vi "Keithley2200series_2_dose.vi"() -> ()   [LabVIEW 2010]
uses:
  <vilib>/Utility/file.llb/Write To Spreadsheet File (string).vi
  C:/Users/rad/Desktop/Keithley 2200 Series Power Supplies Ver 1.2 (LV2009)/Keithley 2200 Series/Keithley 2200 Series.lvlib
panel:
  in  "millisecond multiple":u32
  out "Время,с":dbl
  in  "SEE th 2":dbl
  in  "SEE th 1":dbl
  in  "+ИП2":bool
  out "MEAS 2":string
  in  "Cml set 2":dbl
  in  "Function(0:Voltage) 3":u16(ring) items=["Voltage", "Current"]
  in  "Out set 2":dbl
  in  "VISA resource name 2":refnum<visa-resource-name>
  in  "Cml set":dbl
  in  "Function(0:Voltage) 2":u16(ring) items=["Voltage", "Current"]
  in  "Out set":dbl
  in  "Файл записи замеров":path
  out "MEAS":string
  in  "VISA resource name":refnum<visa-resource-name>
  in  "stop":bool
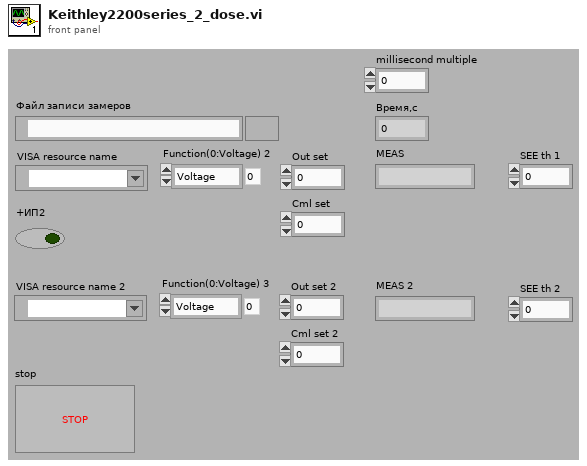
[diagram p1: front panel]
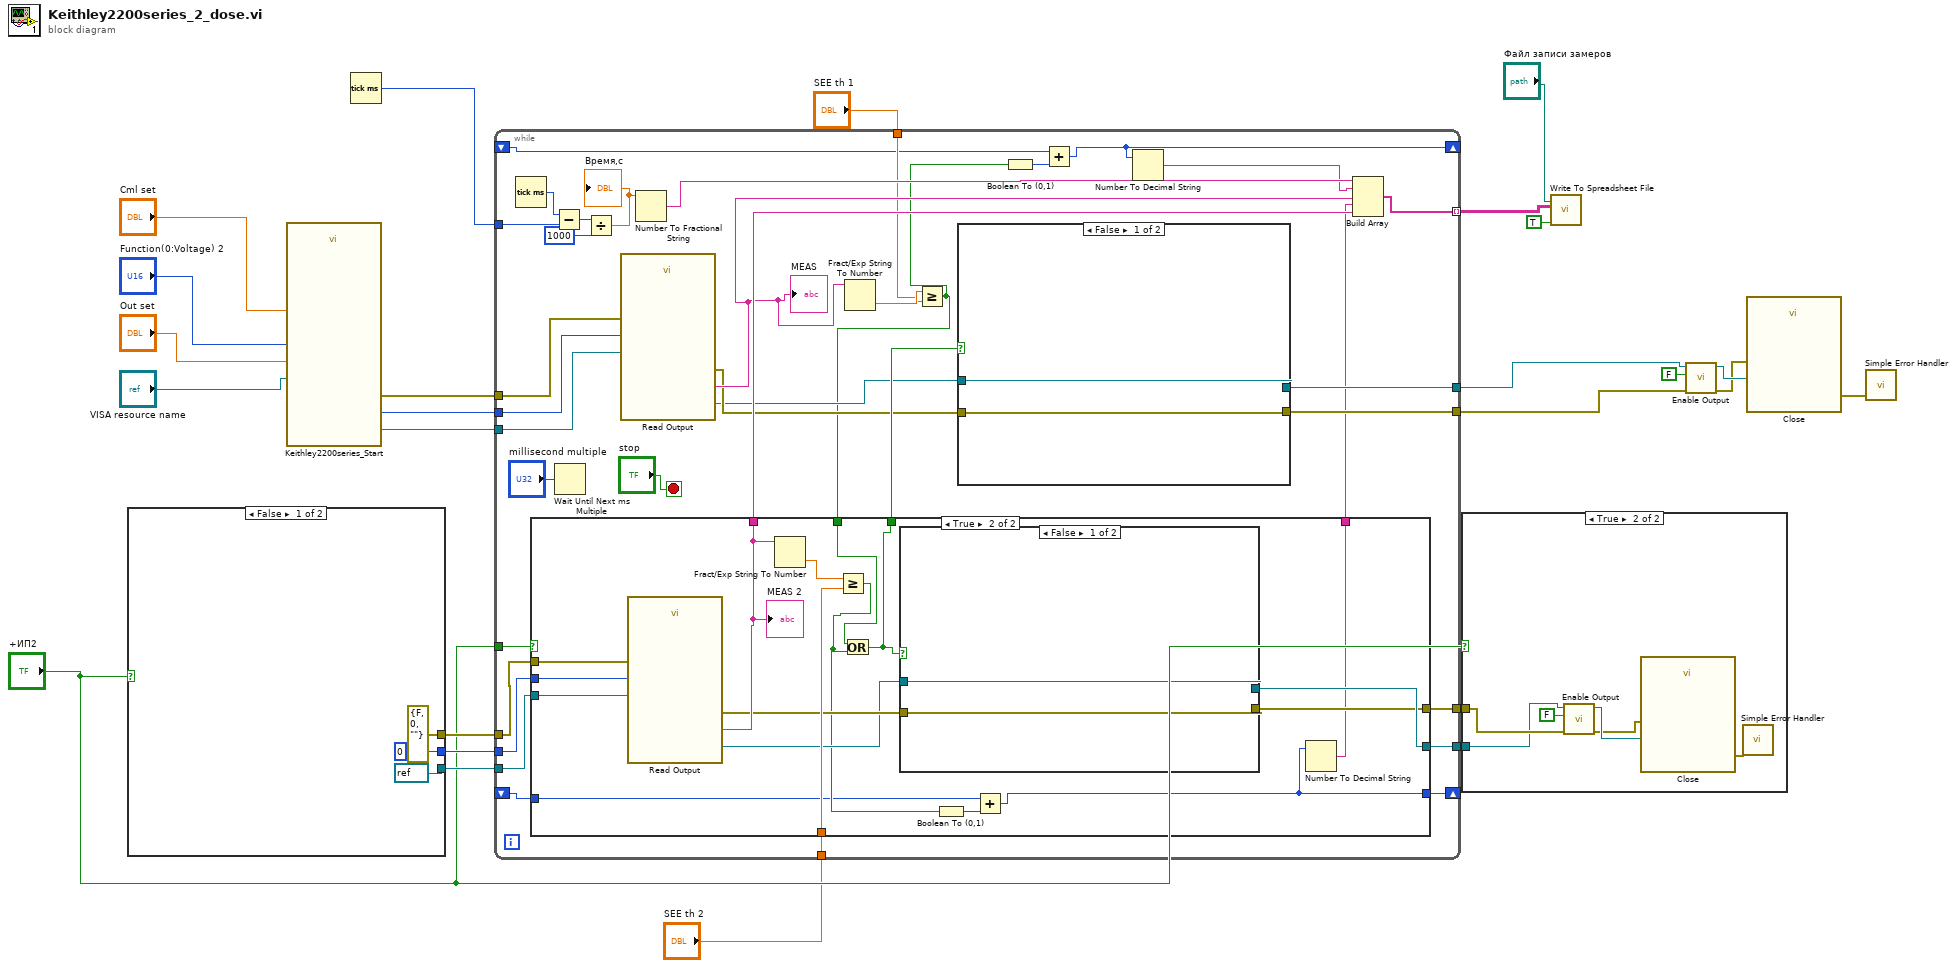
[diagram p0: block diagram]
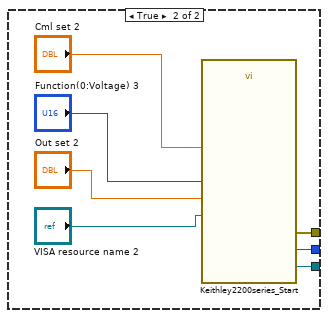
[diagram p3: hidden frame]
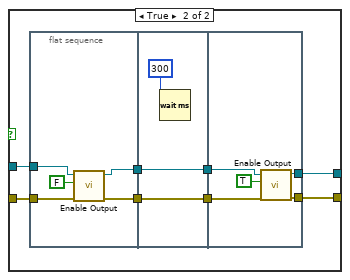
[diagram p4: hidden frame]
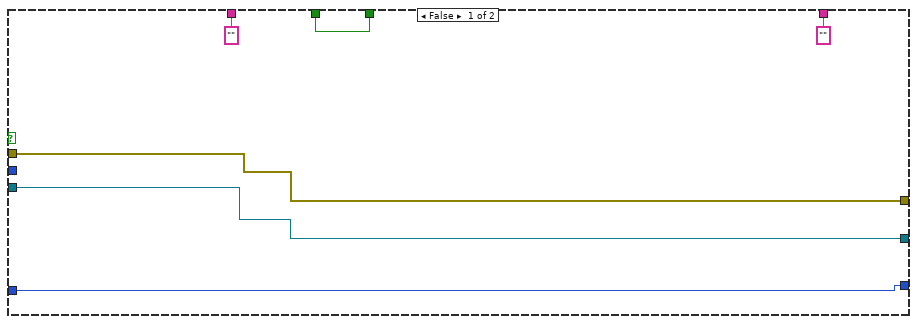
[diagram p5: hidden frame]
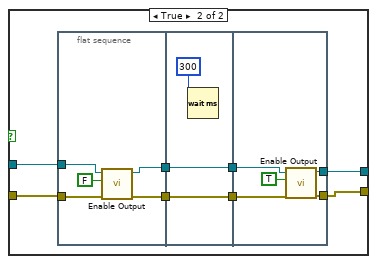
[diagram p6: hidden frame]
diagram:
  n1 = case shown="False" "+ИП2" {
    tunnel: [errorcluster {"status"=FALSE, "code"=0, "source"=""} ("error out 2") w31] -> w12
    tunnel: [0 ("Meas Func") w30] -> w11
    tunnel: [refnum<visa-resource-name> refnum ("VISA out") w29] -> w10
    frame False {
    }
    frame True {
      n2 = call "Keithley2200series_Start.vi"("VISA resource name 2"="VISA resource name 2", "Function(0:Voltage) 3"="Function(0:Voltage) 3", "Out set 2"="Out set 2", "Cml set 2"="Cml set 2") -> ("VISA out"=w29:refnum<visa-resource-name>, "Meas Func"=w30:i32, "error out 2"=w31:errorcluster)  [unwired: 1 in]
    }
  }
  n3 = call "Keithley2200series_Start.vi"("VISA resource name 2"="VISA resource name", "Function(0:Voltage) 3"="Function(0:Voltage) 2", "Out set 2"="Out set", "Cml set 2"="Cml set") -> ("VISA out"=w18:refnum<visa-resource-name>, "Meas Func"=w17:i32, "error out 2"=w16:errorcluster)  [unwired: 1 in]
  n4 = Tick Count (ms)() -> (millisecond timer value=w25:u32)
  n5 = while {
    tunnel: w25 -> [w70]
    tunnel: [w44] -> w24 mode=indexing
    tunnel: w18 -> [w65]
    tunnel: w17 -> [w64]
    tunnel: w16 -> [w63]
    tunnel: [w61] -> w14
    tunnel: [w60] -> w13
    tunnel: w12 -> [w59]
    tunnel: w11 -> [w58]
    tunnel: w10 -> [w57]
    tunnel: "+ИП2" -> [w56]
    tunnel: "SEE th 1" -> [w52]
    tunnel: "SEE th 2" -> [w51]
    tunnel: [w47] -> w3
    tunnel: [w46] -> w2
    shift-right: [w41] -> _
    shift-left: _ -> [w43]
    shift-right: [w38] -> _
    shift-left: _ -> [w39]
    stop <- "stop" stop-if-true
    n6 = Tick Count (ms)() -> (millisecond timer value=w71:u32)
    n7 = Subtract(x=w71, y=w70) -> (x-y=w68:u32)
    n8 = Wait Until Next ms Multiple(millisecond multiple="millisecond multiple") -> ()  [unwired: 1 out]
    n9 = Divide(x=w68, y=u32 1000) -> (x/y=w66:dbl)
    "Время,с" <- w66
    n10 = call "Read Output.vi"("VISA resource name"=w65, "Measurement Function (0:Voltage)"=w64, "error in (no error)"=w63) -> ("VISA resource name out"=w48:refnum<visa-resource-name>, "Measurement"=w54:string, "error out"=w49:errorcluster)  [unwired: 10 in]
    "MEAS" <- w54
    n11 = Number To Fractional String(number=w66) -> (F-format string=w69:string)  [unwired: 3 in]
    n12 = Fract/Exp String To Number(string=w54) -> (number=w53:dbl)  [unwired: 3 in, 1 out]
    n13 = Greater Or Equal?(x=w53, y=w52) -> (x >= y?=w42:bool)
    n14 = case shown="True" w56 {
      tunnel: [w100 w106] -> w61
      tunnel: [w99 w107] -> w60
      tunnel: ["" ("Measurement") w114] -> w55
      tunnel: w59 -> [w100 w117]
      tunnel: w58 -> [_ w116]
      tunnel: w57 -> [w99 w115]
      tunnel: w51 -> [_ w113]
      tunnel: w42 -> [w97 w111]
      tunnel: [w97 w110] -> w50
      tunnel: w39 -> [w96 w103]
      tunnel: [w96 w102] -> w38
      tunnel: ["" w101] -> w37
      frame False {
      }
      frame True {
        n15 = call "Read Output.vi"("VISA resource name"=w115, "Measurement Function (0:Voltage)"=w116, "error in (no error)"=w117) -> ("VISA resource name out"=w108:refnum<visa-resource-name>, "Measurement"=w114:string, "error out"=w109:errorcluster)  [unwired: 10 in]
        "MEAS 2" <- w114
        n16 = Fract/Exp String To Number(string=w114) -> (number=w112:dbl)  [unwired: 3 in, 1 out]
        n17 = Greater Or Equal?(x=w112, y=w113) -> (x >= y?=w104:bool)
        n18 = Or(x=w111, y=w104) -> (x .or. y?=w110:bool)
        n19 = case shown="False" w110 {
          tunnel: w109 -> [w118 w123]
          tunnel: w108 -> [w119 w122]
          tunnel: [w119 w121] -> w107
          tunnel: [w118 w120] -> w106
          frame False {
          }
          frame True {
            n20 = flat-sequence {
              tunnel: w123 -> [w131]
              tunnel: w122 -> [w130]
              tunnel: [w129] -> w127
              tunnel: [w128] -> w126
              tunnel: [w134] -> w125
              tunnel: w127 -> [w134]
              tunnel: [w133] -> w124
              tunnel: w126 -> [w133]
              tunnel: w125 -> [w139]
              tunnel: w124 -> [w138]
              tunnel: [w137] -> w121
              tunnel: [w136] -> w120
              frame #0 {
                n21 = call "Enable Output.vi"("error in (no error)"=w131, "Enable Output (T: Enable)"=FALSE, "VISA resource name"=w130) -> ("error out"=w128:errorcluster, "VISA resource name out"=w129:refnum<visa-resource-name>)  [unwired: 7 in]
              }
              frame #1 {
                n22 = Wait (ms)(milliseconds to wait=u32 300) -> ()  [unwired: 1 out]
              }
              frame #2 {
                n23 = call "Enable Output.vi"("error in (no error)"=w138, "Enable Output (T: Enable)"=TRUE, "VISA resource name"=w139) -> ("error out"=w136:errorcluster, "VISA resource name out"=w137:refnum<visa-resource-name>)  [unwired: 7 in]
              }
            }
          }
        }
        n24 = Boolean To (0,1)(Boolean=w104) -> (0, 1=w105:i16)
        n25 = Add(x=w103, y=w105) -> (x+y=w102:i16)
        n26 = Number To Decimal String(number=w102) -> (decimal integer string=w101:string)  [unwired: 1 in]
      }
    }
    n27 = case shown="False" w50 {
      tunnel: w49 -> [w72 w81]
      tunnel: w48 -> [w73 w80]
      tunnel: [w73 w75] -> w47
      tunnel: [w72 w74] -> w46
      frame False {
      }
      frame True {
        n28 = flat-sequence {
          tunnel: w81 -> [w85]
          tunnel: w80 -> [w84]
          tunnel: [w83] -> w78
          tunnel: [w82] -> w76
          tunnel: [w88] -> w79
          tunnel: w78 -> [w88]
          tunnel: [w87] -> w77
          tunnel: w76 -> [w87]
          tunnel: w79 -> [w93]
          tunnel: w77 -> [w92]
          tunnel: [w91] -> w75
          tunnel: [w90] -> w74
          frame #0 {
            n29 = call "Enable Output.vi"("error in (no error)"=w85, "Enable Output (T: Enable)"=FALSE, "VISA resource name"=w84) -> ("error out"=w82:errorcluster, "VISA resource name out"=w83:refnum<visa-resource-name>)  [unwired: 7 in]
          }
          frame #1 {
            n30 = Wait (ms)(milliseconds to wait=u32 300) -> ()  [unwired: 1 out]
          }
          frame #2 {
            n31 = call "Enable Output.vi"("error in (no error)"=w92, "Enable Output (T: Enable)"=TRUE, "VISA resource name"=w93) -> ("error out"=w90:errorcluster, "VISA resource name out"=w91:refnum<visa-resource-name>)  [unwired: 7 in]
          }
        }
      }
    }
    n32 = Boolean To (0,1)(Boolean=w42) -> (0, 1=w45:i16)
    n33 = Add(x=w43, y=w45) -> (x+y=w41:i16)
    n34 = Number To Decimal String(number=w41) -> (decimal integer string=w40:string)  [unwired: 1 in]
    n35 = Build Array(w69, w40, w54, w37, w55) -> (w44:string[])
  }
  n36 = case shown="True" "+ИП2" {
    tunnel: w14 -> [_ w144]
    tunnel: w13 -> [_ w143]
    frame False {
    }
    frame True {
      n37 = call "Enable Output.vi"("error in (no error)"=w144, "Enable Output (T: Enable)"=FALSE, "VISA resource name"=w143) -> ("error out"=w141:errorcluster, "VISA resource name out"=w142:refnum<visa-resource-name>)  [unwired: 7 in]
      n38 = call "Close.vi"("error in (no error)"=w141, "VISA resource name"=w142) -> ("error out"=w146:errorcluster)  [unwired: 9 in]
      n39 = call <vilib>:"Simple Error Handler.vi"("error in (no error)"=w146) -> ()  [unwired: 4 in, 5 out]
    }
  }
  n40 = call-poly <vilib>:"Write To Spreadsheet File.vi"("append to file? (new file:F)"=TRUE, "2D data"=w24, "file path (dialog if empty)"="Файл записи замеров") -> ()  [unwired: 5 in, 1 out]
  n41 = call "Enable Output.vi"("error in (no error)"=w2, "Enable Output (T: Enable)"=FALSE, "VISA resource name"=w3) -> ("error out"=w7:errorcluster, "VISA resource name out"=w8:refnum<visa-resource-name>)  [unwired: 7 in]
  n42 = call "Close.vi"("error in (no error)"=w7, "VISA resource name"=w8) -> ("error out"=w15:errorcluster)  [unwired: 9 in]
  n43 = call <vilib>:"Simple Error Handler.vi"("error in (no error)"=w15) -> ()  [unwired: 4 in, 5 out]
